vi "StatusStripDemo.vi"() -> ()   [LabVIEW 2013]
uses:
  StatusStripClass/StatusStripClass.lvclass
  System.Windows.Forms
panel:
  in  "停止":bool
  in  "StatusStrip":refnum<k24>(container)
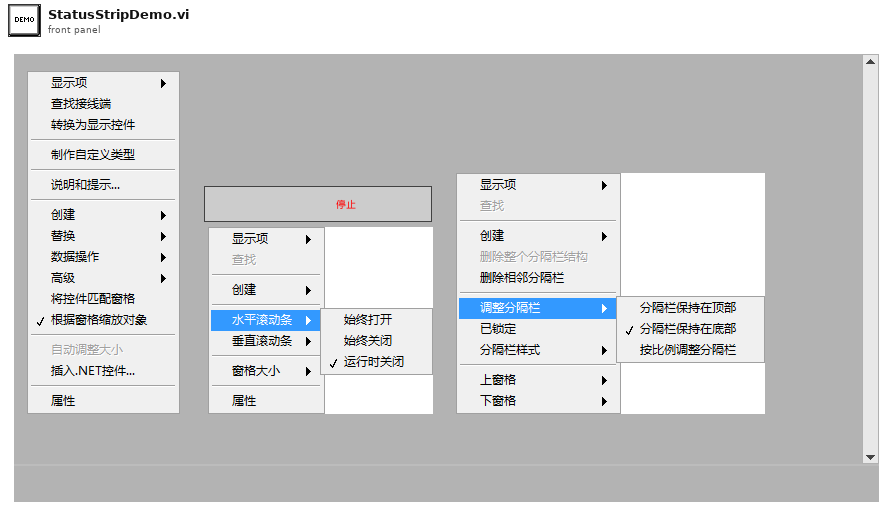
[diagram p1: front panel]
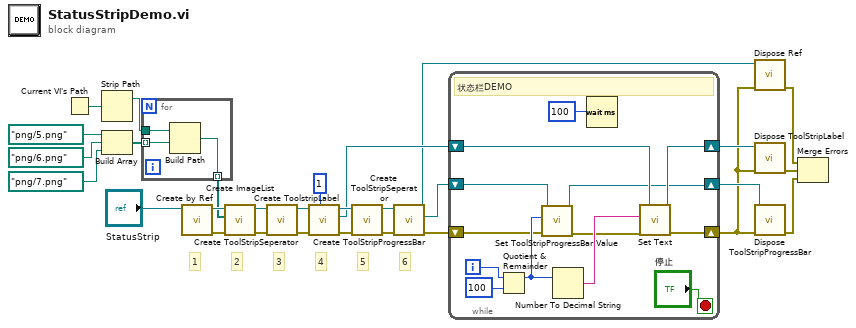
[diagram p0: block diagram]
diagram:
  # "6"
  # "5"
  # "4"
  # "3"
  # "2"
  # "1"
  n1 = Current VI's Path() -> (path=w5:path)
  n2 = Strip Path(path=w5) -> (stripped path=w3:path)  [unwired: 1 out]
  n3 = Build Array(path "png/5.png", path "png/6.png", path "png/7.png") -> (w4:path[])
  n4 = for {
    tunnel: w4 -> [w31] mode=indexing
    tunnel: w3 -> [w32]
    tunnel: [w30] -> w2 mode=indexing
    n5 = Build Path(base path=w32, name or relative path=w31) -> (appended path=w30:path)
  }
  n6 = call "Create by Ref.vi"("StatusStrip"="StatusStrip") -> ("error out"=w27:errorcluster, "StatusStripClass 输出"=w26:refnum<class "StatusStripClass.lvclass">)  [unwired: 8 in]
  n7 = call "Create ImageList.vi"("error in (no error)"=w27, "ImgPath"=w2, "StatusStripClass 输入"=w26) -> ("error out"=w24:errorcluster, "StatusStripClass 输出"=w25:refnum<class "StatusStripClass.lvclass">)  [unwired: 7 in]
  n8 = call "Create ToolStripSeperator.vi"("error in (no error)"=w24, "StatusStripClass 输入"=w25) -> ("error out"=w22:errorcluster, "StatusStripClass 输出"=w23:refnum<class "StatusStripClass.lvclass">)  [unwired: 8 in]
  n9 = call "Create ToolstripLabel.vi"("ImageIndex"=1, "error in (no error)"=w22, "StatusStripClass 输入"=w23) -> ("error out"=w20:errorcluster, "ToolStripLabel 输出"=w17:refnum<class "ToolStripLabel.lvclass">, "StatusStripClass 输出"=w21:refnum<class "StatusStripClass.lvclass">)  [unwired: 6 in]
  n10 = call "Create ToolStripSeperator.vi"("error in (no error)"=w20, "StatusStripClass 输入"=w21) -> ("error out"=w18:errorcluster, "StatusStripClass 输出"=w19:refnum<class "StatusStripClass.lvclass">)  [unwired: 8 in]
  n11 = call "Create ToolStripProgressBar.vi"("error in (no error)"=w18, "StatusStripClass 输入"=w19) -> ("error out"=w15:errorcluster, "ToolStripProgressBar 输出"=w16:refnum<class "ToolStripProgressBar.lvclass">, "StatusStripClass 输出"=w10:refnum<class "StatusStripClass.lvclass">)  [unwired: 7 in]
  n12 = while {
    shift-right: [w43] -> w14
    shift-left: w17 -> [w44]
    shift-right: [w34] -> w9
    shift-left: w15 -> [w38]
    shift-right: [w36] -> w13
    shift-left: w16 -> [w37]
    i -> [w41]
    stop <- "停止" stop-if-true
    # "状态栏DEMO"
    n13 = Quotient & Remainder(x=w41, y=100) -> (x-y*floor(x/y)=w39:i32)  [unwired: 1 out]
    n14 = call "Set ToolStripProgressBar Value.vi"("error in (no error)"=w38, "Value"=w39, "ToolStripProgressBar 输入"=w37) -> ("error out"=w35:errorcluster, "ToolStripProgressBar 输出"=w36:refnum<class "ToolStripProgressBar.lvclass">)  [unwired: 7 in]
    n15 = Number To Decimal String(number=w39) -> (decimal integer string=w40:string)  [unwired: 1 in]
    n16 = Wait (ms)(milliseconds to wait=u32 100 ("等待时间（毫秒）")) -> ()  [unwired: 1 out]
    n17 = call "Set Text.vi"("error in (no error)"=w35, "Text"=w40, "ToolStripLabel 输入"=w44) -> ("error out"=w34:errorcluster, "ToolStripLabel 输出"=w43:refnum<class "ToolStripLabel.lvclass">)  [unwired: 7 in]
  }
  n18 = call "Dispose Ref.vi"("error in (no error)"=w9, "StatusStripClass 输入"=w10) -> ("error out"=w8:errorcluster)  [unwired: 9 in]
  n19 = call "Dispose ToolStripLabel.vi"("error in (no error)"=w9, "ToolStripLabel 输入"=w14) -> ("error out"=w12:errorcluster)  [unwired: 8 in, 1 out]
  n20 = call "Dispose ToolStripProgressBar.vi"("error in (no error)"=w9, "ToolStripProgressBar 输入"=w13) -> ("error out"=w11:errorcluster)  [unwired: 9 in]
  n21 = Merge Errors(w8, w12, w11) -> ()  [unwired: 1 out]
